vi "nudgePositive.vi"(11 "Min in":T1) -> (3 "Min out":T1)   [LabVIEW 2013]
uses:
  AutoManualNumber.ctl
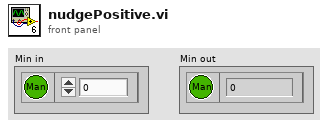
[diagram p1: front panel]
types:
  T1 = typedef "AutoManualNumber.ctl" = cluster{"Auto":bool, "Value":dbl}
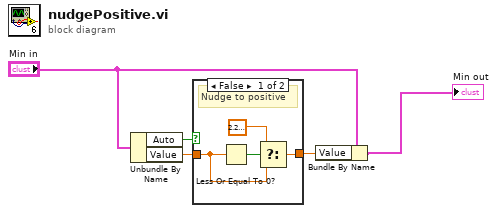
[diagram p0: block diagram]
diagram:
  n1 = Unbundle By Name("Min in") -> ("Auto"=w2:bool, "Value"=w1:dbl)
  n2 = case shown="False" w2 {
    tunnel: w1 -> [w8 w10]
    tunnel: [w6 w10] -> w4
    frame False {
      # "Nudge to positive"
      n3 = Less Or Equal To 0?(x=w8) -> (x <= 0?=w9:bool)
      n4 = Select(t=2.220446049250313e-16, s=w9, f=w8) -> (s? t:f=w6:dbl)
    }
    frame True {
    }
  }
  n5 = Bundle By Name(cluster="Min in", "Value"=w4) -> (→"Min out":T1)
